vi "Version Cluster to String.vi"(8 "error in (no error)":errorcluster, 11 "version":T1) -> (0 "error out":errorcluster, 3 "version string":string)   [LabVIEW 2019, in "DSF System Explorer.lvlib"]
uses:
  DSF System Explorer.lvlib
  DSF Core.lvlibp/Typedefs/DSF Version Info.ctl
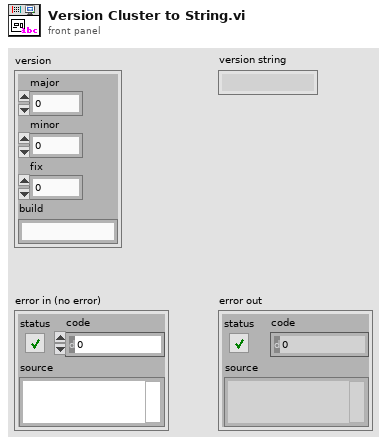
[diagram p1: front panel]
types:
  T1 = typedef "DSF Core.lvlibp/DSF Version Info.ctl" = cluster{"major":u32, "minor":u32, "fix":u32, "build":string}
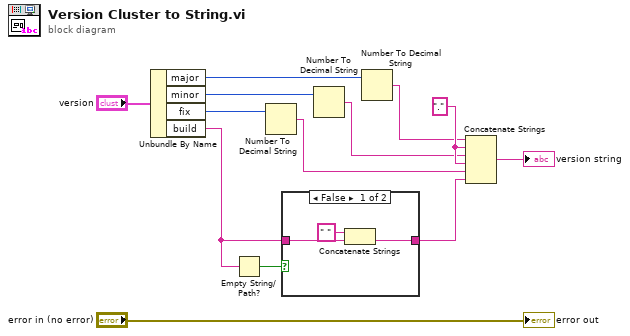
[diagram p0: block diagram]
diagram:
  w9 = "."
  n1 = Unbundle By Name("version") -> ("major"=w12:u32, "minor"=w11:u32, "fix"=w10:u32, "build"=w5:string)
  n2 = Empty String/Path?(string/path=w5) -> (empty?=w4:bool)
  n3 = Number To Decimal String(number=w10) -> (decimal integer string=w6:string)  [unwired: 1 in]
  n4 = case shown="False" w4 {
    tunnel: w5 -> [w15 w17]
    tunnel: [w14 w17] -> w3
    frame False {
      n5 = Concatenate Strings(" " ("string"), w15) -> (w14:string)
    }
    frame True {
    }
  }
  n6 = Number To Decimal String(number=w11) -> (decimal integer string=w7:string)  [unwired: 1 in]
  n7 = Number To Decimal String(number=w12) -> (decimal integer string=w8:string)  [unwired: 1 in]
  n8 = Concatenate Strings(w8, w9, w7, w9, w6, w3) -> (→"version string":string)
  "error out" <- "error in (no error)"
